vi "CreateIntegerArray.vi"(10 "Input Parameters":T1) -> (2 "Output Array":i32[](array[numeric]))   [LabVIEW 2015]
doc: "CreateIntegerArray that creates an array with given minimum, maximum and number of points. It also should be able to select between linear and logarithmic spacing. It should always have integer outputs."
uses:
  <vilib>/imath/engines/lvmath2/RunTimeEngine/Managers/WorkSpace/UID Generator.vi
  <vilib>/imath/engines/lvmath2/RunTimeSupport/NIMS_Complex To Real.vi
  <instcachedir>/0/NIMS_Complex To Real_01315F44AA8B4CE79FEF95AE999DC25E.lvgen/NIMS_Complex To Real_01315F44AA8B4CE79FEF95AE999DC25E_001.vi
  <vilib>/imath/engines/lvmath2/RunTimeEngine/BuiltInFunctions/logramp/NIMS_logramp.vi
  <vilib>/imath/engines/lvmath2/RunTimeEngine/RunTimeType/NIMS_RunTimeType_From StrictType (excl LVString).vi
  <instcachedir>/0/NIMS_RunTimeType_From StrictType (excl LVString)_EB1C38A9BC5048DA9ABDA8F781E54D21.lvgen/NIMS_RunTimeType_From StrictType (excl LVString)_EB1C38A9BC5048DA9ABDA8F781E54D21_000.vi
  <vilib>/imath/engines/lvmath2/RunTimeEngine/ErrorHandling/NIMS_Create Error From Enums.vi
  <vilib>/imath/engines/lvmath2/RunTimeEngine/LocalVariableDefStatement/MC_LocalVariableDefStatement_Display.vi
  <vilib>/imath/engines/lvmath2/RunTimeEngine/BuiltInFunctions/linramp/NIMS_linramp.vi
  <vilib>/imath/engines/lvmath2/RunTimeEngine/Managers/SymbolTable/Clear UID.vi
  <vilib>/imath/engines/lvmath2/RunTimeEngine/NodeEndStatement/NIMS_NodeEndStatement_Output.vi
  <instcachedir>/0/NIMS_NodeEndStatement_Output_53EC0D466D134D7ABD903AC30B43404B.lvgen/NIMS_NodeEndStatement_Output_53EC0D466D134D7ABD903AC30B43404B_005.vi
  <vilib>/imath/engines/lvmath2/RunTimeEngine/ErrorHandling/NIMS_Finalize Error.vi
  <vilib>/imath/engines/lvmath2/RunTimeEngine/Managers/SymbolTable/NIMS_WorkSpace.lvlib
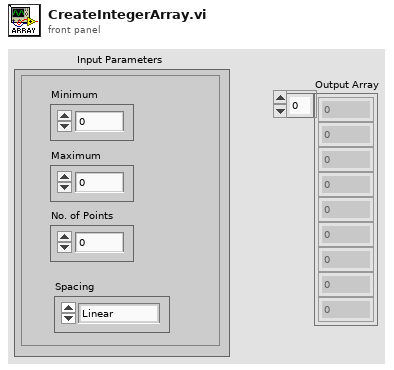
[diagram p1: front panel]
types:
  T1 = cluster{"Minimum":i32, "Maximum":i32, "No. of Points":i32, "Spacing":enum16{"Linear", "Logarithmic"}}
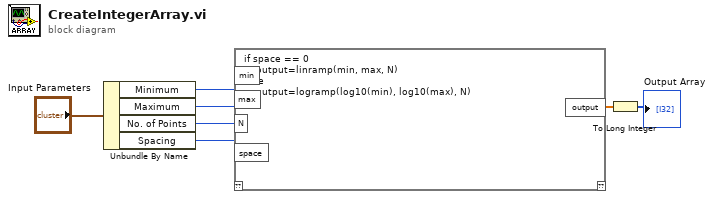
[diagram p0: block diagram]
diagram:
  n1 = Unbundle By Name("Input Parameters") -> ("Minimum"=w3:i32, "Maximum"=w4:i32, "No. of Points"=w5:i32, "Spacing"=w6:enum16{"Linear", "Logarithmic"})
  n2 = mathscript code="if space == 0\n    output=linramp(min, max, N)\nelse \n    output=logramp(log10(min), log10(max), N)\nend"("min"=w3, "max"=w4, "N"=w5, "space"=w6) -> ("output"=w2:dbl[])  [unwired: 1 in, 1 out]
  n3 = To Long Integer(number=w2) -> (32bit integer=→"Output Array":i32[])
